vi "acqBeep.vi"(8 "error in":errorcluster) -> (0 "error out":errorcluster)   [LabVIEW 2020]
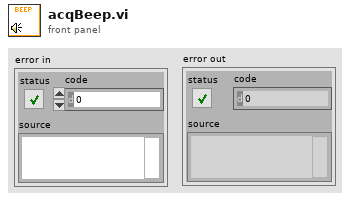
[diagram p1: front panel]
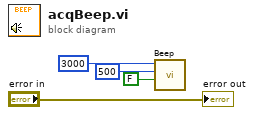
[diagram p0: block diagram]
diagram:
  n1 = call <vilib>:"Beep.vi"("use system alert? (T)"=FALSE, "duration (msec)"=u32 500, "frequency (Hz)"=u32 3000) -> ()  [unwired: 9 in]
  "error out" <- "error in"
